vi "StartStop.vi"(8 "error in (no error)":errorcluster, 10 "Start/stop":bool, 11 "Generador de Funciones in":refnum<class "Generador de Funciones.lvclass">) -> (0 "error out":errorcluster, 3 "Generador de Funciones out":refnum<class "Generador de Funciones.lvclass">)   [LabVIEW 2020, in "Generador de Funciones.lvlib" / "Generador de Funciones.lvclass"]
uses:
  Generador de Funciones.lvclass
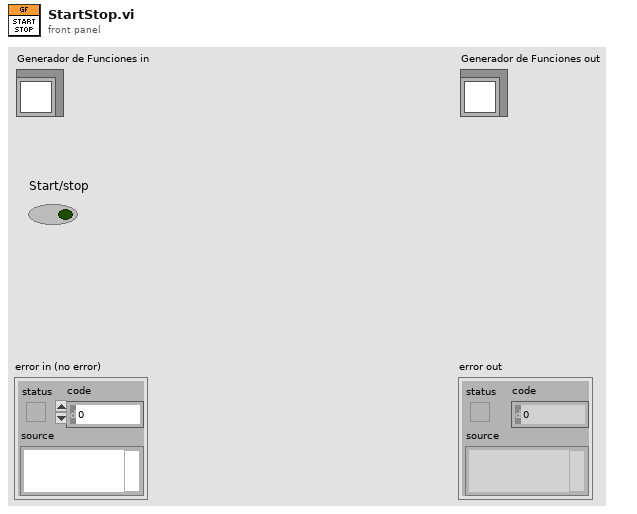
[diagram p1: front panel]
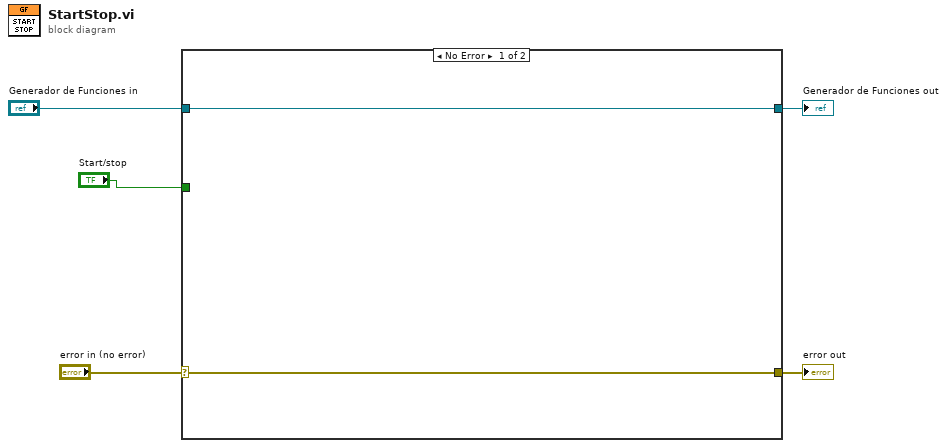
[diagram p0: block diagram]
diagram:
  n1 = case shown="No Error" "error in (no error)" {
    selector: "error in (no error)" -> [w6 w9]
    tunnel: [w6 w9] -> w4
    tunnel: [w7 w8] -> w2
    tunnel: "Generador de Funciones in" -> [w7 w8]
    tunnel: "Start/stop" -> [_ _]
    frame No Error {
    }
    frame Error {
    }
  }
  "error out" <- w4
  "Generador de Funciones out" <- w2
